vi "ReadSub(SubVI).vi"(8 "error in":errorcluster) -> (0 "error out":errorcluster, 3 "Output":string)   [LabVIEW 2014]
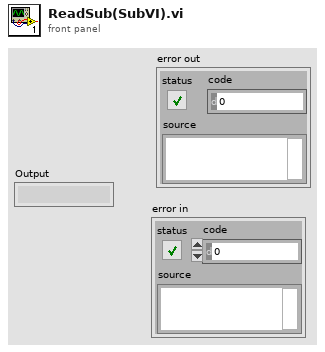
[diagram p1: front panel]
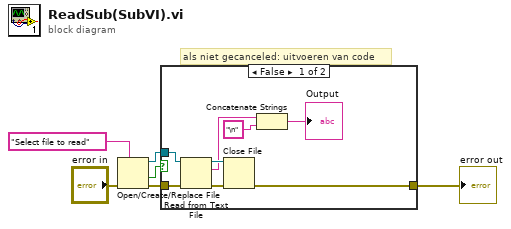
[diagram p0: block diagram]
diagram:
  # "als niet gecanceled: uitvoeren van code"
  n1 = Open/Create/Replace File(error in="error in", prompt="Select file to read") -> (refnum out=w5:refnum<file>, cancelled=w4:bool, error out=w6:errorcluster)  [unwired: 4 in]
  n2 = case shown="False" w4 {
    tunnel: w5 -> [w14 _]
    tunnel: w6 -> [w11 w15]
    tunnel: [w7 w15] -> w2
    frame False {
      n3 = Read from Text File(file (use dialog)=w14, error in=w11) -> (refnum out=w13:refnum<file>, text=w9:string, error out=w12:errorcluster)  [unwired: 2 in, 1 out]
      n4 = Close File(refnum=w13, error in=w12) -> (error out=w7:errorcluster)  [unwired: 1 out]
      n5 = Concatenate Strings(w9, "\n") -> (→"Output":string)
    }
    frame True {
    }
  }
  "error out" <- w2
